vi "op-selector.vi"(9 "Prev AO":T1, 10 "Channel":T2={"Operation"=0, "Input A"=0, "Output - LO"=0.0, "Output - HI"=0.0, "Inputs"=[0, 0, 0, 0], "Output Values"=[0.0, 0.0, 0.0, 0.0, 0.0], "Num. Inputs"=4, "Set Point"=0.0, "Inv."=[FALSE, FALSE, FALSE, FALSE], "Inv. A"=FALSE, "Inv. B"=FALSE, "Input B"=0} {"Input B" items=["DIO0", "DIO1", "DIO2", "DIO3", "DIO4", "DIO5", "DIO6", "DIO7", "DIO8", "DIO9", "DIO10", "DIO11", "DIO12", "DIO13", "DIO14", "DIO15", "DIO16", "DIO17", "DIO18", "DIO19", "DIO20", "DIO21", "DIO22", "DIO23", "DIO24", "DIO25", "DIO26", "DIO27", "DIO28", "DIO29", "DIO30", "DIO31", "FALSE"]; "Input A" items=["DIO0", "DIO1", "DIO2", "DIO3", "DIO4", "DIO5", "DIO6", "DIO7", "DIO8", "DIO9", "DIO10", "DIO11", "DIO12", "DIO13", "DIO14", "DIO15", "DIO16", "DIO17", "DIO18", "DIO19", "DIO20", "DIO21", "DIO22", "DIO23", "DIO24", "DIO25", "DIO26", "DIO27", "DIO28", "DIO29", "DIO30", "DIO31", "FALSE"]; "Inputs" items=["DIO0", "DIO1", "DIO2", "DIO3", "DIO4", "DIO5", "DIO6", "DIO7", "DIO8", "DIO9", "DIO10", "DIO11", "DIO12", "DIO13", "DIO14", "DIO15", "DIO16", "DIO17", "DIO18", "DIO19", "DIO20", "DIO21", "DIO22", "DIO23", "DIO24", "DIO25", "DIO26", "DIO27", "DIO28", "DIO29", "DIO30", "DIO31", "FALSE"]; "Operation" items=["OFF", "Constant", "Bool - Basic Switch", "Bool - AND Switch", "Bool - OR Switch", "Custom - Comp Basic Switch", "Custom - 461nm Freq."]}, 11 "Digital Input Value Array":bool[](array[boolean])=[FALSE, FALSE, FALSE, FALSE, FALSE, FALSE, FALSE, FALSE, FALSE, FALSE, FALSE, FALSE, FALSE, FALSE, FALSE, FALSE, FALSE, FALSE, FALSE, FALSE, FALSE, FALSE, FALSE, FALSE, FALSE, FALSE, FALSE, FALSE, FALSE, FALSE, FALSE, FALSE]) -> (1 "New AO":T1)   [LabVIEW 2016]
uses:
  op_ctrl_element.ctl
  DIO_selector.ctl
  output_value.ctl
panel:
  # "Constant Operation Control"
  # "Boolean Operation Control"
  # "Custom Operation Controls"
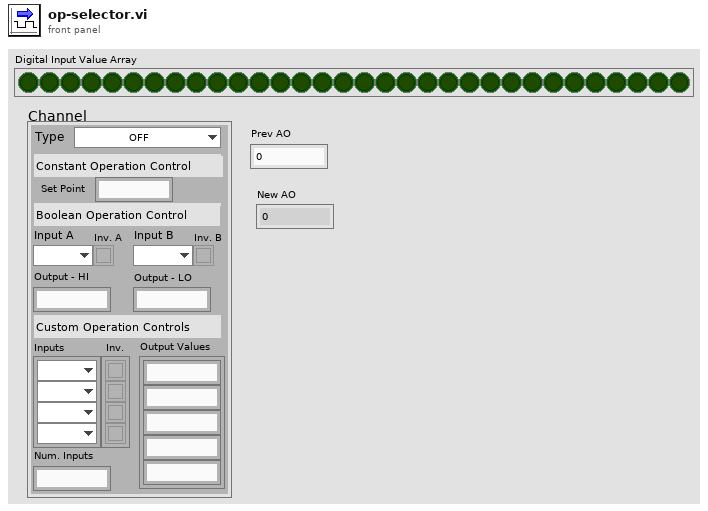
[diagram p1: front panel]
types:
  T1 = typedef "output_value.ctl" = fxp<+/-,20,5>
  T2 = typedef "op_ctrl_element.ctl" = cluster{"Operation":i16, "Input A":T3, "Output - LO":T1, "Output - HI":T1, "Inputs":T3[], "Output Values":T1[], "Num. Inputs":i32, "Set Point":T1, "Inv.":bool[], "Inv. A":bool, "Inv. B":bool, "Input B":T3}
  T3 = typedef "DIO_selector.ctl" = i32
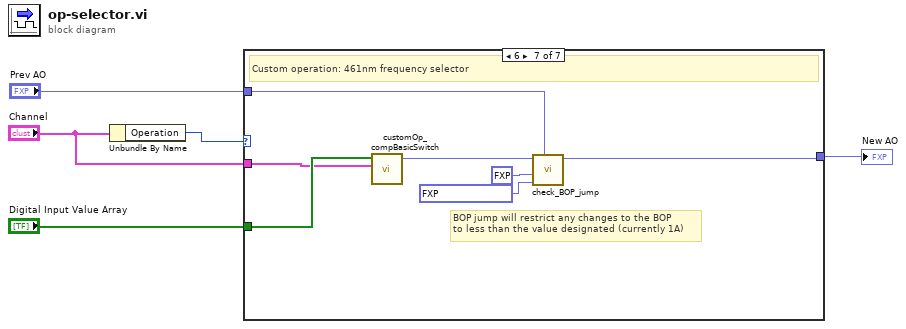
[diagram p0: block diagram]
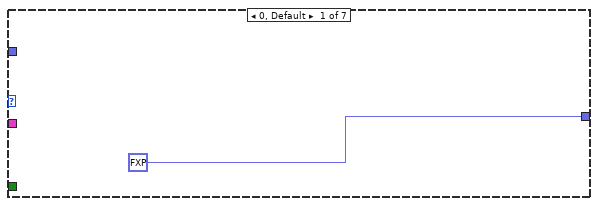
[diagram p2: hidden frame]
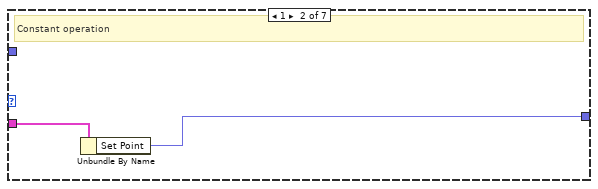
[diagram p3: hidden frame]
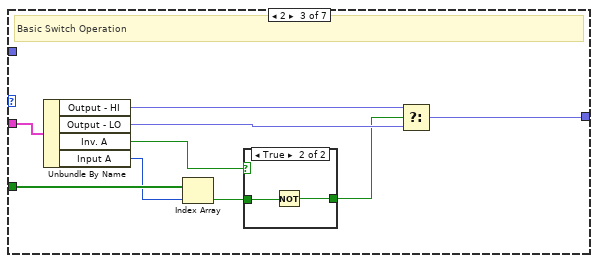
[diagram p4: hidden frame]
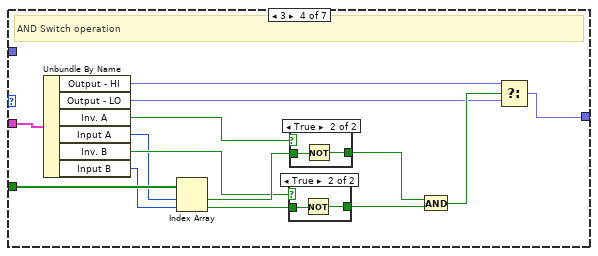
[diagram p6: hidden frame]
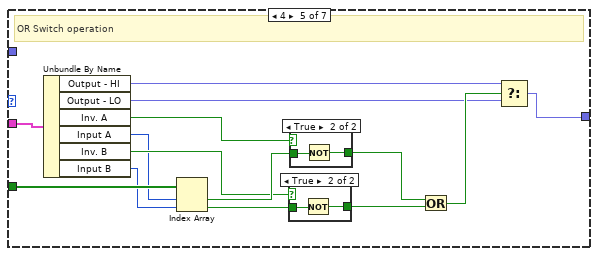
[diagram p9: hidden frame]
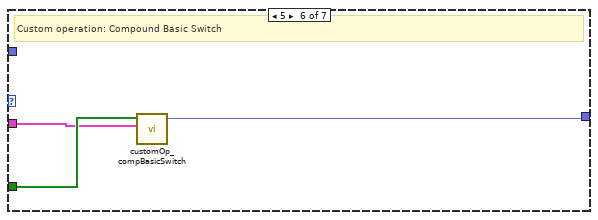
[diagram p12: hidden frame]
diagram:
  n1 = Unbundle By Name("Channel") -> ("Operation"=w4:i16)
  n2 = case shown="6" w4 {
    tunnel: [fxp<+,20,5> 0.0 w7 w14 w30 w50 w61 w67] -> w1
    tunnel: "Channel" -> [_ w8 w17 w34 w54 w62 w69]
    tunnel: "Digital Input Value Array" -> [_ _ w13 w29 w49 w63 w70]
    tunnel: "Prev AO" -> [_ _ _ _ _ _ w66]
    frame 0, Default {
    }
    frame 1 {
      # "Constant operation"
      n3 = Unbundle By Name(w8) -> ("Set Point"=w7:T1)
    }
    frame 2 {
      # "Basic Switch Operation"
      n4 = Unbundle By Name(w17) -> ("Output - HI"=w15:T1, "Output - LO"=w16:T1, "Inv. A"=w11:bool, "Input A"=w12:T3)
      n5 = Index Array(array=w13, index=w12) -> (element=w10:bool)
      n6 = case shown="True" w11 {
        tunnel: w10 -> [w18 w20]
        tunnel: [w18 w19] -> w9
        frame False {
        }
        frame True {
          n7 = Not(x=w20) -> (.not. x?=w19:bool)
        }
      }
      n8 = Select(t=w15, s=w9, f=w16) -> (s? t:f=w14:T1)
    }
    frame 3 {
      # "AND Switch operation"
      n9 = Unbundle By Name(w34) -> ("Output - HI"=w32:T1, "Output - LO"=w31:T1, "Inv. A"=w23:bool, "Input A"=w24:T3, "Inv. B"=w25:bool, "Input B"=w26:T3)
      n10 = Index Array(array=w29, index #1=w24, index #2=w26) -> (element #1=w27:bool, element #2=w28:bool)
      n11 = case shown="True" w25 {
        tunnel: w28 -> [w38 w40]
        tunnel: [w38 w39] -> w21
        frame False {
        }
        frame True {
          n12 = Not(x=w40) -> (.not. x?=w39:bool)
        }
      }
      n13 = case shown="True" w23 {
        tunnel: w27 -> [w35 w37]
        tunnel: [w35 w36] -> w22
        frame False {
        }
        frame True {
          n14 = Not(x=w37) -> (.not. x?=w36:bool)
        }
      }
      n15 = And(x=w22, y=w21) -> (x .and. y?=w33:bool)
      n16 = Select(t=w32, s=w33, f=w31) -> (s? t:f=w30:T1)
    }
    frame 4 {
      # "OR Switch operation"
      n17 = Unbundle By Name(w54) -> ("Output - HI"=w52:T1, "Output - LO"=w51:T1, "Inv. A"=w43:bool, "Input A"=w44:T3, "Inv. B"=w45:bool, "Input B"=w46:T3)
      n18 = Index Array(array=w49, index #1=w44, index #2=w46) -> (element #1=w47:bool, element #2=w48:bool)
      n19 = case shown="True" w45 {
        tunnel: w48 -> [w58 w60]
        tunnel: [w58 w59] -> w41
        frame False {
        }
        frame True {
          n20 = Not(x=w60) -> (.not. x?=w59:bool)
        }
      }
      n21 = case shown="True" w43 {
        tunnel: w47 -> [w55 w57]
        tunnel: [w55 w56] -> w42
        frame False {
        }
        frame True {
          n22 = Not(x=w57) -> (.not. x?=w56:bool)
        }
      }
      n23 = Or(x=w42, y=w41) -> (x .or. y?=w53:bool)
      n24 = Select(t=w52, s=w53, f=w51) -> (s? t:f=w50:T1)
    }
    frame 5 {
      # "Custom operation: Compound Basic Switch"
      n25 = call "customOp_compBasicSwitch.vi"("Channel"=w62, "Digital Input Value Array"=w63) -> ("AO Out"=w61:fxp<+/-,20,5>)  [unwired: 9 in]
    }
    frame 6 {
      # "BOP jump will restrict any changes to the BOP\nto less than the value designated (currently 1A)"
      # "Custom operation: 461nm frequency selector"
      n26 = call "customOp_compBasicSwitch.vi"("Channel"=w69, "Digital Input Value Array"=w70) -> ("AO Out"=w68:fxp<+/-,20,5>)  [unwired: 9 in]
      n27 = call "check_BOP_jump.vi"("Prev AO"=w66, "Increment Amount"=fxp<+/-,20,5> 0.0050048828125, "BOP jump limit"=fxp<+/-,20,5> 1.5, "AO to Check"=w68) -> ("AO Out"=w67:fxp<+/-,21,6>)  [unwired: 7 in]
    }
  }
  "New AO" <- w1
